vi "Analyze Event Step 1 (Non-40MHz).vi"(7 "measure settings.<user name>":T4, 8 "register bus":T2={"Speed"="Speed", "Crank Angle"="Crank Angle", "Cycle Angle"="Cycle Angle", "Crank Count"="Crank Count", "Cycle Count"="Cycle Count", "1.25 MHz Counter"="1.25 MHz Counter", "Crank Rollover"="Crank Rollover", "Cycle Rollover"="Cycle Rollover", "shared settings"={"start"=0.0, "stuck limit"=0.0}} {"shared settings"."start" format="%#.15g"}, 10 "event":bool) -> (3 "windowed event data":T1)   [LabVIEW 2015, in "Engine Simulation Toolkit.lvlib" / "ECU Event Timing.lvlib"]
uses:
  ECU Event Timing.lvlib
  Measure Settings.ctl
  APU/Register Bus.ctl
  APU/Shared Settings.ctl
  Windowed Event Data.ctl
  <vilib>/Utility/error.llb/Clear Errors.vi
  <vilib>/rvi/Emulation/niFpgaSctlEmulationGetInTimedLoop.vi
  <vilib>/rvi/DataTransferAndStorage/Container/Common/niFpgaContainerExecOnDevCompGetState.vi
  <vilib>/rvi/Emulation/niFpgaEmulationIsFPGAContextNoSignature.vi
  <vilib>/rvi/DataTransferAndStorage/Container/Common/niFpgaContainerGetUniqueNameForEmu.vi
  <vilib>/rvi/Memory/Memory_Emulation/niFpgaMemoryEmulationCacheClearOnFirstRun.vi
  <vilib>/rvi/Memory/Memory_Emulation/nirvimemoryEmulationManagerCache_MakeExclusive.vi
  <vilib>/rvi/Memory/Memory_Emulation/niFpgaMemoryEmulationValidateCache.vi
  <vilib>/rvi/Memory/Memory_Emulation/nirvimemoryEmulationManagerCache_InsertValue.vi
  <vilib>/rvi/Memory/Memory_Emulation/nirvimemoryEmulationManagerCache_ReleaseExclusive.vi
  <vilib>/rvi/Memory/Memory_Emulation/nirvimemoryEmulationManagerCache_GetValue.vi
  <vilib>/rvi/Memory/Memory_Emulation/nirvimemoryEmulationManagerCache_SetValue.vi
  <vilib>/rvi/Emulation/niFpgaProcessEmulError.vi
  <vilib>/rvi/DataTransferAndStorage/Container/XNode/niFpgaContainer.xnode
  <vilib>/rvi/DataTransferAndStorage/Register/Emulation/niFpgaRegisterEmulationRefIn.vi
  Engine Simulation Toolkit.lvlib
  APU/APU.lvlib
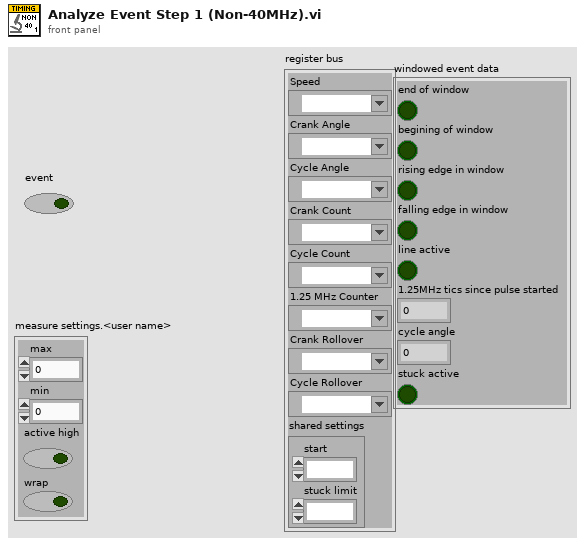
[diagram p1: front panel]
types:
  T1 = typedef "Engine Simulation Toolkit.lvlib/ECU Event Timing.lvlib/Windowed Event Data.ctl" = cluster{"end of window":bool, "begining of window":bool, "rising edge in window":bool, "falling edge in window":bool, "line active":bool, "1.25MHz tics since pulse started":fxp<+,18,18>, "cycle angle":u16, "stuck active":bool}
  T2 = typedef "Engine Simulation Toolkit.lvlib/APU.lvlib/Register Bus.ctl" = cluster{"Speed":refnum<k21>, "Crank Angle":refnum<k21>, "Cycle Angle":refnum<k21>, "Crank Count":refnum<k21>, "Cycle Count":refnum<k21>, "1.25 MHz Counter":refnum<k21>, "Crank Rollover":refnum<k21>, "Cycle Rollover":refnum<k21>, "shared settings":T3}
  T3 = typedef "Engine Simulation Toolkit.lvlib/APU.lvlib/Shared Settings.ctl" = cluster{"start":fxp<+,17,17>, "stuck limit":fxp<+,18,18>}
  T4 = typedef "Engine Simulation Toolkit.lvlib/ECU Event Timing.lvlib/Measure Settings.ctl" = cluster{"max":u16, "min":u16, "active high":bool, "wrap":bool}
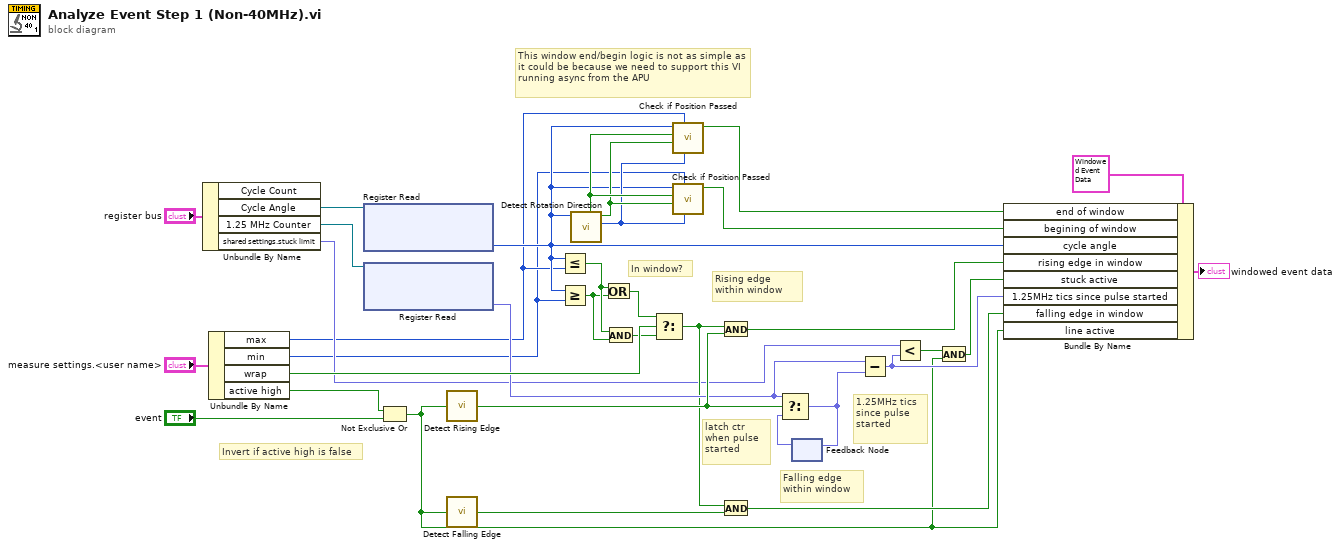
[diagram p0: block diagram]
diagram:
  # "This window end/begin logic is not as simple as it could be because we need to support this VI running async from the APU"
  # "latch ctr when pulse started"
  # "1.25MHz tics since pulse started"
  # "Falling edge within window"
  # "Rising edge within window"
  # "Invert if active high is false"
  # "In window?"
  n1 = Unbundle By Name("register bus") -> ("Cycle Angle"=w32:refnum<k21>, "1.25 MHz Counter"=w23:refnum<k21>, "shared settings.stuck limit"=w9:fxp<+,18,18>)  [unwired: 1 out]
  n2 = Unbundle By Name("measure settings.<user name>") -> ("max"=w4:u16, "min"=w3:u16, "wrap"=w26:bool, "active high"=w29:bool)
  n3 = xnode ("Register Read")("Register In"=w32) -> ("Data"=w5:u16)  [unwired: 1 out]
  n4 = xnode ("Register Read")("Register In"=w23) -> ("Data"=w20:fxp<+,18,18>)  [unwired: 1 out]
  n5 = Not Exclusive Or(1:"event", 2:w29) -> (0:w10:bool)
  n6 = call "Detect Rising Edge.vi"("signal"=w10) -> ("edge detected"=w22:bool)  [unwired: 14 in]
  n7 = call "Detect Falling Edge.vi"("signal"=w10) -> ("edge detected"=w30:bool)  [unwired: 14 in]
  n8 = Less Or Equal?(x=w5, y=w4) -> (x <= y?=w28:bool)
  n9 = Greater Or Equal?(x=w5, y=w3) -> (x >= y?=w27:bool)
  n10 = call "Detect Rotation Direction.vi"("position"=w5) -> ("previous position (n-1)"=w6:u16, "rotated forward or stopped"=w7:bool, "cycle wrapped"=w8:bool)  [unwired: 8 in]
  n11 = Or(x=w28, y=w27) -> (x .or. y?=w25:bool)
  n12 = And(x=w28, y=w27) -> (x .and. y?=w24:bool)
  n13 = Select(t=w25, s=w26, f=w24) -> (s? t:f=w18:bool)
  n14 = call "Check if Position Passed.vi"("previous position (n-1)"=w6, "trigger position"=w4, "rotated forward"=w7, "cycle wrapped"=w8, "position"=w5) -> ("trigger"=w1:bool)  [unwired: 6 in]
  n15 = call "Check if Position Passed.vi"("previous position (n-1)"=w6, "trigger position"=w3, "rotated forward"=w7, "cycle wrapped"=w8, "position"=w5) -> ("trigger"=w2:bool)  [unwired: 6 in]
  n16 = And(x=w18, y=w22) -> (x .and. y?=w16:bool)
  n17 = And(x=w18, y=w30) -> (x .and. y?=w15:bool)
  n18 = feedback #1() -> (w21:fxp<+,18,18>)  [unwired: 1 in]
  n19 = Select(t=w20, s=w22, f=w21) -> (s? t:f=w19:fxp<+,18,18>)
  n20 = feedback-in #1(w19) -> ()
  n21 = Subtract(x=w20, y=w19) -> (x-y=w13:fxp<+,18,18>)
  n22 = Less?(x=w9, y=w13) -> (x < y?=w12:bool)
  n23 = And(x=w12, y=w10) -> (x .and. y?=w11:bool)
  n24 = Bundle By Name(cluster=T1 {"end of window"=FALSE, "begining of window"=FALSE, "rising edge in window"=FALSE, "falling edge in window"=FALSE, "line active"=FALSE, "1.25MHz tics since pulse started"=0.0, "cycle angle"=0, "stuck active"=FALSE} ("Windowed event data"), "end of window"=w1, "begining of window"=w2, "cycle angle"=w5, "rising edge in window"=w16, "stuck active"=w11, "1.25MHz tics since pulse started"=w13, "falling edge in window"=w15, "line active"=w10) -> (→"windowed event data":T1)
